vi "Omron_DM_Write.vi"(4 "Command":string="WR", 6 "Number of Data":u16=1 min=1 max=30 format="%04.0f", 7 "Beginning Words":u16 max=9999 format="%04.0f", 8 "error in":errorcluster, 9 "Write Data":i16[](array[numeric]) max=9999 format="%04.0f", 10 "Unit No.":u8 max=31 format="%02.0f", 11 "COM in":refnum<visa-resource-name>) -> (0 "error out":errorcluster, 3 "COM out":refnum<visa-resource-name>)   [LabVIEW 2015]
panel:
  out "连接的字符串":string
  out "Response":string
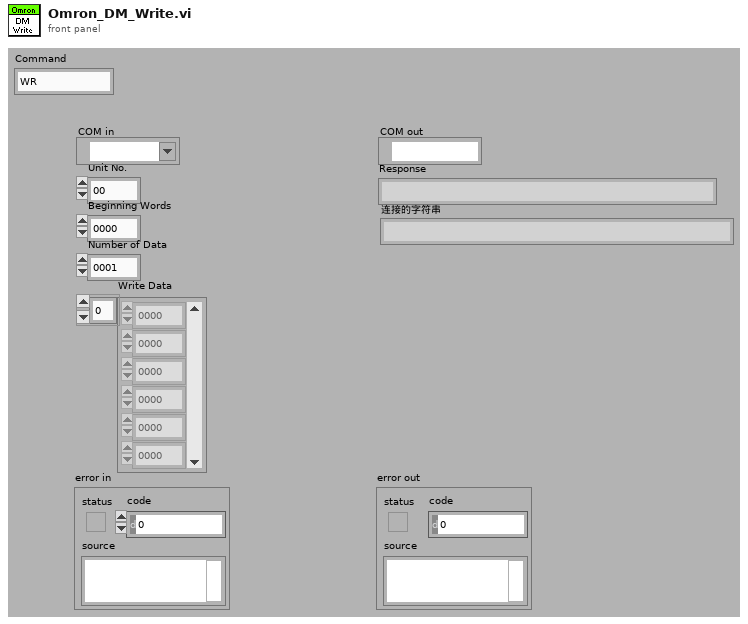
[diagram p1: front panel]
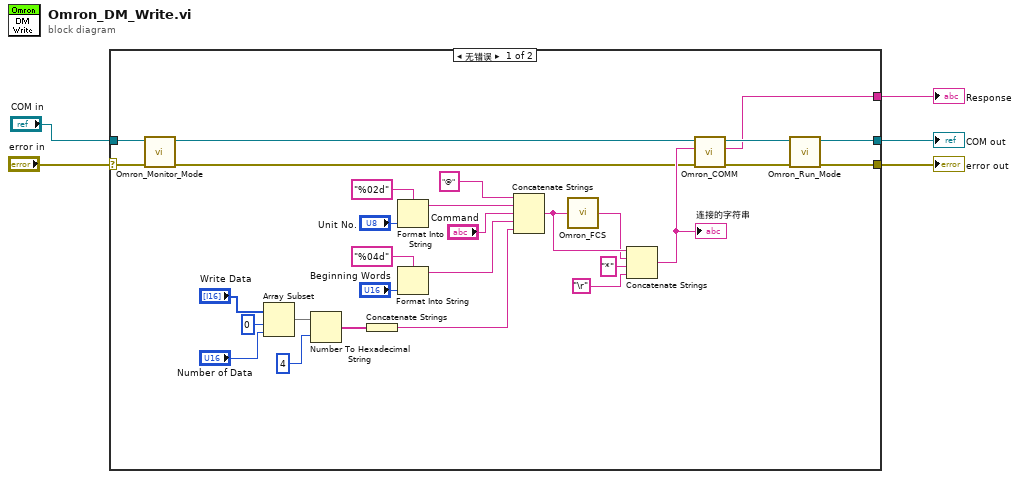
[diagram p0: block diagram]
diagram:
  n1 = case shown="无错误" "error in" {
    selector: "error in" -> [w13 w35]
    tunnel: "COM in" -> [w15 w36]
    tunnel: [w12 w36] -> w2
    tunnel: [w10 w35] -> w1
    tunnel: [w17 _] -> w5
    frame No Error {
      n2 = call "Omron_Monitor_Mode.vi"("error in"=w13, "COM in"=w15) -> ("error out"=w14:errorcluster, "COM out"=w16:refnum<visa-resource-name>)  [unwired: 8 in]
      n3 = Array Subset(array="Write Data", index=0, length="Number of Data") -> (w9:i16[])
      n4 = Number To Hexadecimal String(1:i16 4 ("width (-)"), 2:w9) -> (0:w7:string[])
      n5 = Concatenate Strings(w7) -> (w6:string)
      n6 = Format Into String(format string="%02d", "Unit No.") -> (resulting string=w31:string)  [unwired: 2 in, 1 out]
      n7 = Format Into String(format string="%04d", "Beginning Words") -> (resulting string=w27:string)  [unwired: 2 in, 1 out]
      n8 = Concatenate Strings("@" ("Command"), w31, "Command", w27, w6) -> (w26:string)
      n9 = call "Omron_FCS.vi"("Command"=w26) -> ("FCS"=w25:string)
      n10 = Concatenate Strings(w26, w25, "*" ("string"), "\r") -> (w22:string)
      "连接的字符串" <- w22
      n11 = call "Omron_COMM.vi"("error in"=w14, "Write data"=w22, "COM in"=w16) -> ("error out"=w11:errorcluster, "Receive data"=w17:string, "COM out"=w21:refnum<visa-resource-name>)  [unwired: 6 in]
      n12 = call "Omron_Run_Mode.vi"("error in"=w11, "COM in"=w21) -> ("error out"=w10:errorcluster, "COM out"=w12:refnum<visa-resource-name>)  [unwired: 8 in]
    }
    frame Error {
    }
  }
  "COM out" <- w2
  "error out" <- w1
  "Response" <- w5
